vi "GetSensorData.vi"(8 "Error In":errorcluster, 11 "Sensor id":string) -> (0 "Error Out":errorcluster, 2 "Data Out":cluster{"Dates":timestamp[], "Values":dbl[]})   [LabVIEW 2020]
doc: "This VI use GET method to get data from specific sensor and convert JSON string to cluster with measure date/time and value."
uses:
  <vilib>/httpClient/LabVIEWHTTPClient.lvlib
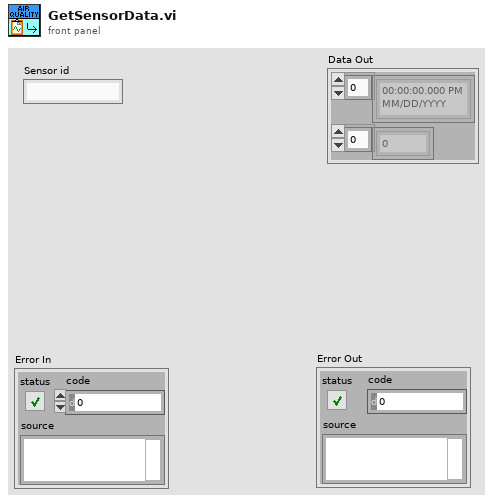
[diagram p1: front panel]
types:
  T1 = cluster{"key":string, "values":cluster{"date":string, "value":dbl}[]}
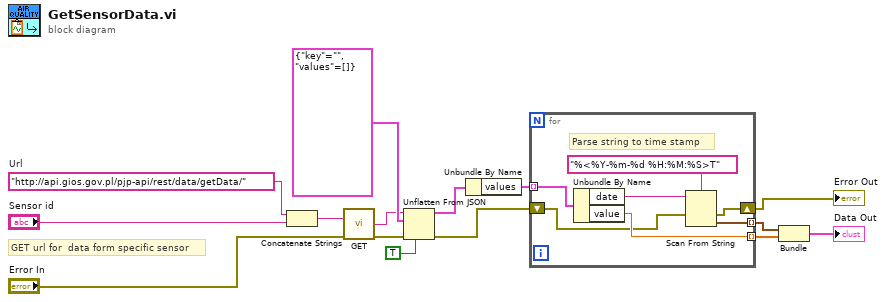
[diagram p0: block diagram]
diagram:
  w14 = "http://api.gios.gov.pl/pjp-api/rest/data/getData/"  # Url
  # "GET url for  data form specific sensor"
  n1 = Concatenate Strings(w14, "Sensor id") -> (w13:string)
  n2 = call <vilib>:"GET.vi"("url"=w13, "error in (no error)"="Error In") -> ("body"=w4:string, "error out"=w8:errorcluster)  [unwired: 10 in, 2 out]
  n3 = Unflatten From JSON(JSON string=w4, type and defaults=T1 {"key"="", "values"=[]}, default null elements? (F)=TRUE, error in (no error)=w8) -> (value=w10:T1, error out=w7:errorcluster)  [unwired: 3 in]
  n4 = Unbundle By Name(w10) -> ("values"=w11:cluster{"date":string, "value":dbl}[])
  n5 = for {
    tunnel: w11 -> [w22] mode=indexing
    tunnel: [w19] -> w3 mode=indexing
    shift-right: [w16] -> w6
    shift-left: w7 -> [w17]
    tunnel: [w21] -> w2 mode=indexing
    # "Parse string to time stamp"
    n6 = Unbundle By Name(w22) -> ("date"=w20:string, "value"=w21:dbl)
    n7 = Scan From String(format string="%<%Y-%m-%d %H:%M:%S>T", input string=w20, error in=w17) -> (error out=w16:errorcluster, output 1=w19:timestamp)  [unwired: 2 in, 2 out]
  }
  "Error Out" <- w6
  n8 = Bundle(w3, w2) -> (→"Data Out":cluster{timestamp[], dbl[]})  [unwired: 1 in]
